vi "RealAction.vi"(11 "TableIn":string[][](array[string])) -> (2 "Step":i32[](array[numeric]), 3 "RealAction":string[][](array[string]))   [LabVIEW 2019]
uses:
  MPC_VirbVision.lvclass
panel:
  out "number":i32[](array[numeric])
  out "deleted portion":string[][](array[string])
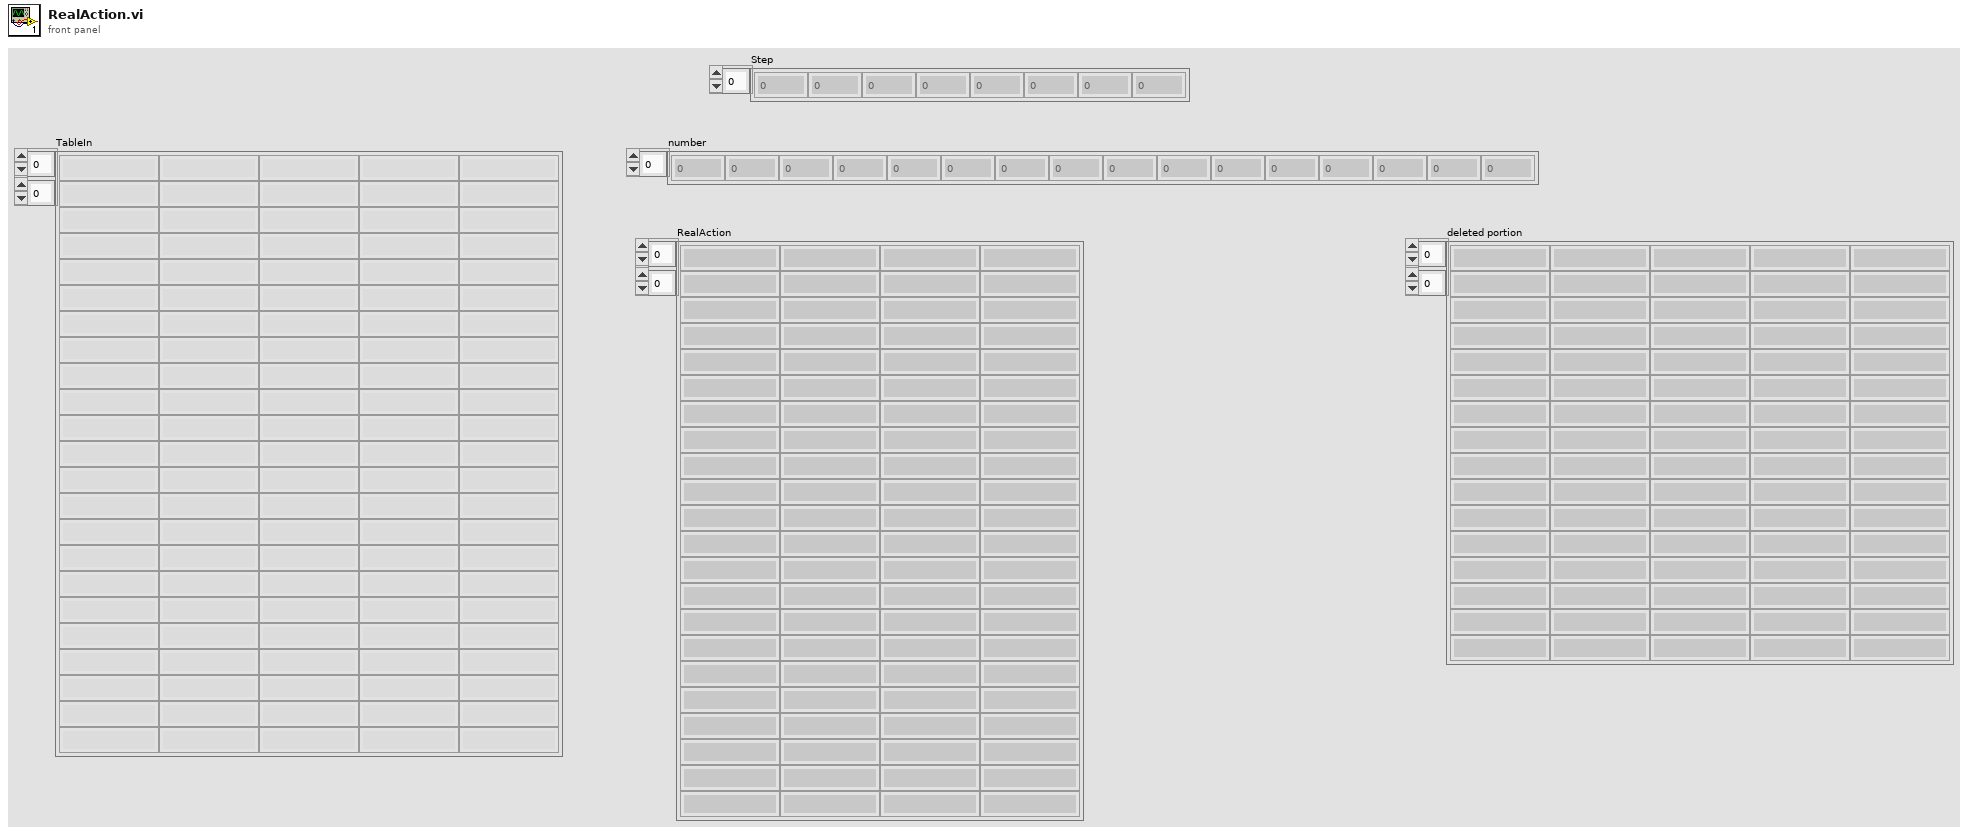
[diagram p1: front panel]
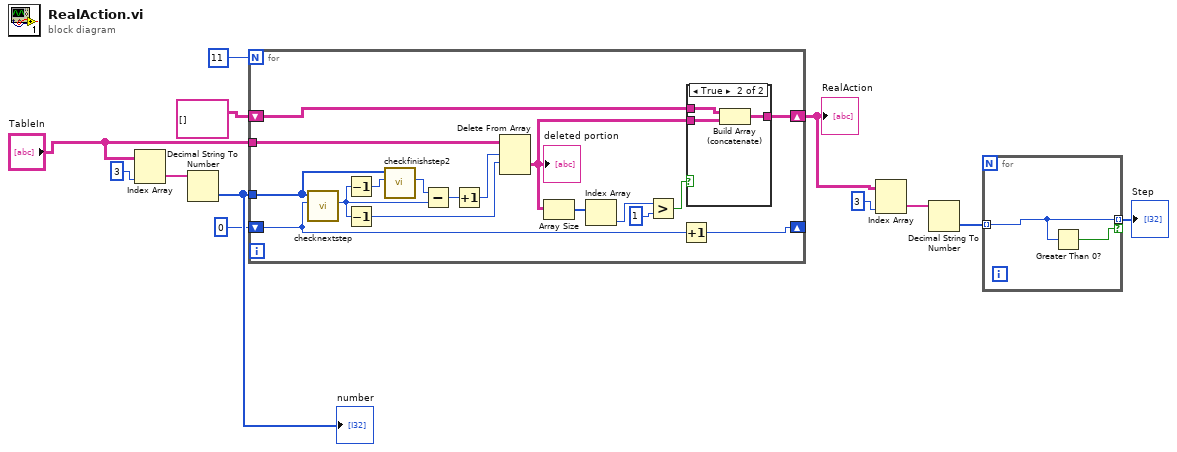
[diagram p0: block diagram]
diagram:
  n1 = Index Array(array="TableIn", index (col)=3 ("disabled index (col)")) -> (element=w11:string[])  [unwired: 1 in]
  n2 = Decimal String To Number(string=w11) -> (number=w10:i32[])  [unwired: 2 in, 1 out]
  "number" <- w10
  n3 = for {
    N: 11 -> [_]
    tunnel: w10 -> [w29]
    shift-right: [w24] -> _
    shift-left: 0 ("Step") -> [w25]
    tunnel: "TableIn" -> [w28]
    shift-right: [w21] -> w3
    shift-left: string[][] [] -> [w20]
    n4 = call "checknextstep.vi"("Step"=w25, "StepNumber"=w29) -> ("Index"=w16:i32)  [unwired: 8 in, 1 out]
    n5 = Decrement(x=w16) -> (x-1=w14:i32)
    n6 = Decrement(x=w16) -> (x-1=w19:i32)
    n7 = call "checkfinishstep2.vi"("Index"=w14, "StepNumber"=w29) -> ("Index"=w27:i32)  [unwired: 7 in, 2 out]
    n8 = Subtract(x=w27, y=w16) -> (x-y=w15:i32)
    n9 = Increment(x=w15) -> (x+1=w13:i32)
    n10 = Delete From Array(array=w28, length=w13, index (row)=w19) -> (deleted portion=w22:string[][])  [unwired: 1 in, 1 out]
    "deleted portion" <- w22
    n11 = Array Size(array=w22) -> (size(s)=w26:i32[])
    n12 = Index Array(array=w26) -> (element=w18:i32)  [unwired: 1 in]
    n13 = Greater?(x=w18, y=1) -> (0:w23:bool)
    n14 = Increment(x=w25) -> (x+1=w24:i32)
    n15 = case shown="True" w23 {
      tunnel: w22 -> [_ w33]
      tunnel: [w30 w32] -> w21
      tunnel: w20 -> [w30 w31]
      frame False {
      }
      frame True {
        n16 = Build Array (concatenate)(w31, w33) -> (w32:string[][])
      }
    }
  }
  "RealAction" <- w3
  n17 = Index Array(array=w3, index (col)=3 ("disabled index (col)")) -> (element=w5:string[])  [unwired: 1 in]
  n18 = Decimal String To Number(string=w5) -> (number=w2:i32[])  [unwired: 2 in, 1 out]
  n19 = for {
    tunnel: w2 -> [w35] mode=indexing
    tunnel: [w35] -> w1 mode=indexing if=w34
    n20 = Greater Than 0?(x=w35) -> (x > 0?=w34:bool)
  }
  "Step" <- w1
